vi "Main.vi"(8 "error in (no error)":errorcluster, 11 "BMCBase in":refnum<class "BMC.lvclass">) -> (0 "error out":errorcluster, 3 "component":refnum<class "BMC.lvclass">)   [LabVIEW 2012, in "BMC.lvclass"]
doc: "Main VI of the component."
uses:
  BMC.lvclass
  Murmex/LabVIEW/Murmex/Murmex/Murmex.lvclass
  Murmex/LabVIEW/Murmex/InitialiseMessage/InitialiseMessage.lvclass
  Murmex/LabVIEW/Murmex/TerminateMessage/TerminateMessage.lvclass
  Murmex/LabVIEW/Murmex/Message/Message.lvclass
  Murmex/LabVIEW/Murmex/ConfigureMessage/ConfigureMessage.lvclass
  Murmex/LabVIEW/Murmex/StartMessage/StartMessage.lvclass
  Murmex/LabVIEW/Murmex/StopMessage/StopMessage.lvclass
  Murmex/LabVIEW/Murmex/Murmex/update_cluster.ctl
  Murmex/LabVIEW/Murmex/Murmex/command_enum.ctl
  Controls/Voltage file.ctl
panel:
  in  "button::quit":bool
  in  "Tab Control":enum32{"Settings", "Debug"}(tab)
  in  "Multi mapping file":path=path "MultiMap.txt"
  in  "Voltage file":T1=path "MultiMap.txt"
  in  "button::configure":bool
  in  "button::start":bool
  in  "button::stop":bool
  in  "command":T2
  in  "button::send":bool
  in  "id":string="myself"
  out "Log":string
  in  "Generic command":string
  out "terminate?":bool
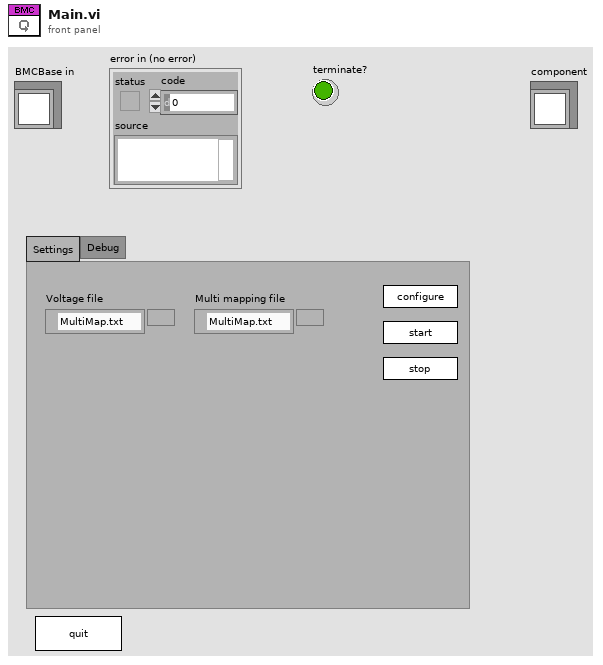
[diagram p1: front panel]
types:
  T1 = typedef "Voltage file.ctl" = path
  T2 = typedef "Murmex.lvclass/command_enum.ctl" = enum16{"null", "initialise", "reset", "terminate", "acknowledge", "update", "inspect", "inform", "proceed", "start", "stop", "fetch", "configure", "generic"}
  T3 = enum8{"Enabled", "Disabled", "Disabled and Grayed Out"}
  T4 = typedef "Murmex.lvclass/update_cluster.ctl" = cluster{"target ID":string, "key chains":string[], "values":variant[]}
  T5 = typedef "Murmex.lvclass/Event type enumerations.ctl" = enum16{"before", "after"}
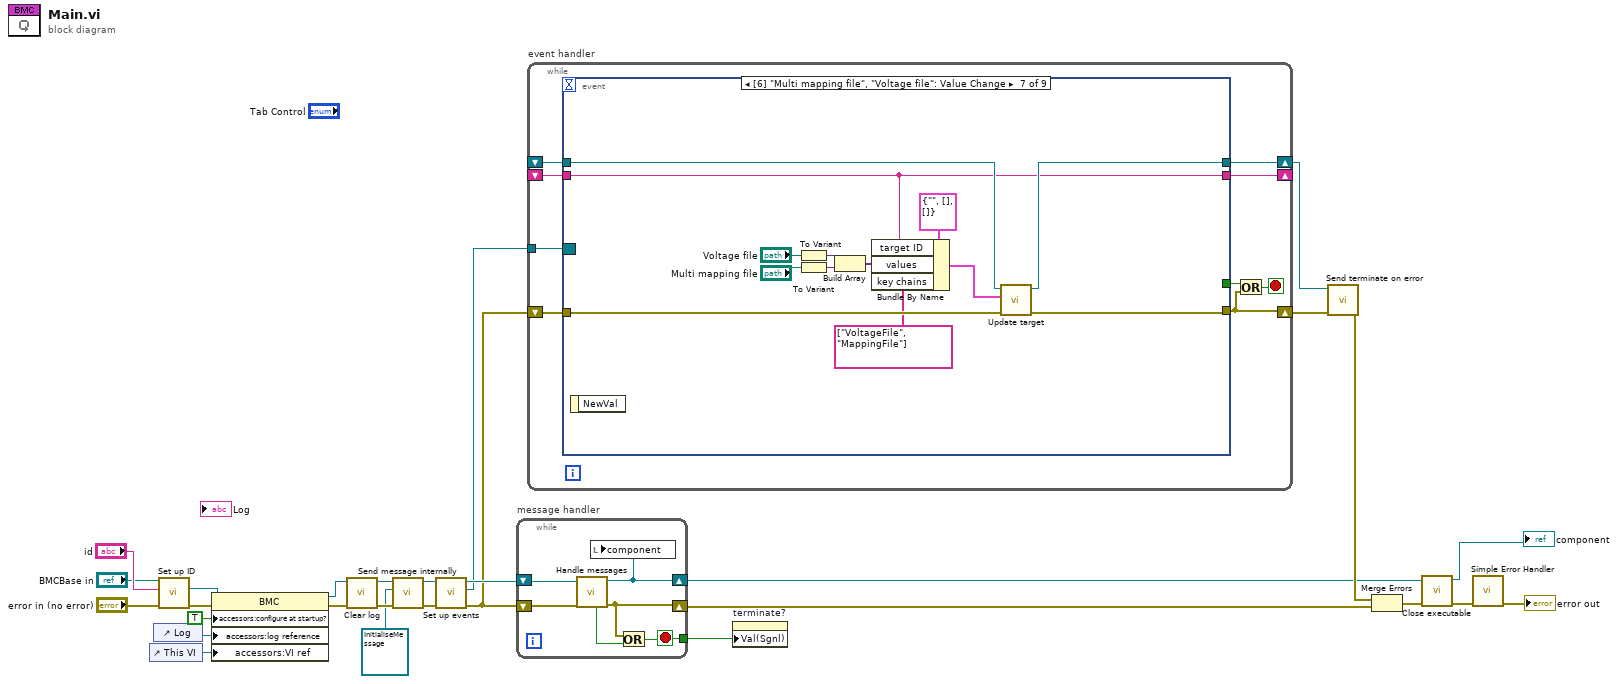
[diagram p0: block diagram]
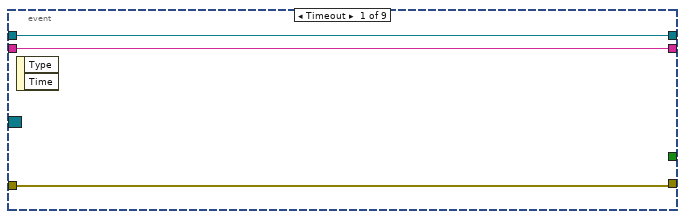
[diagram p2: hidden frame]
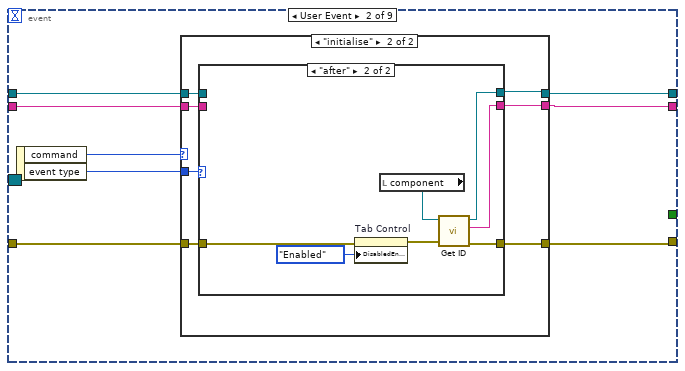
[diagram p3: hidden frame]
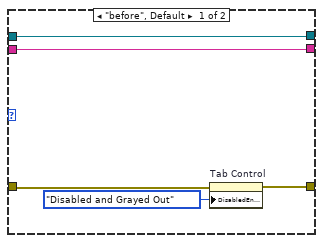
[diagram p5: hidden frame]
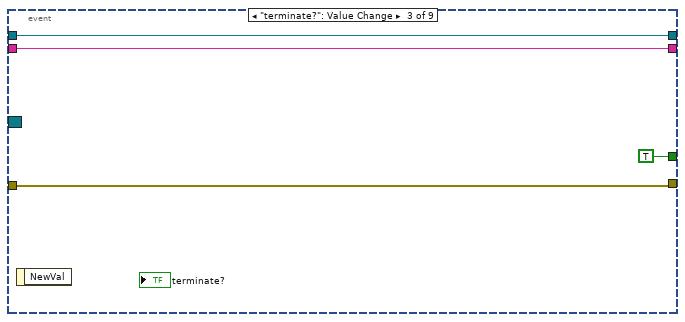
[diagram p6: hidden frame]
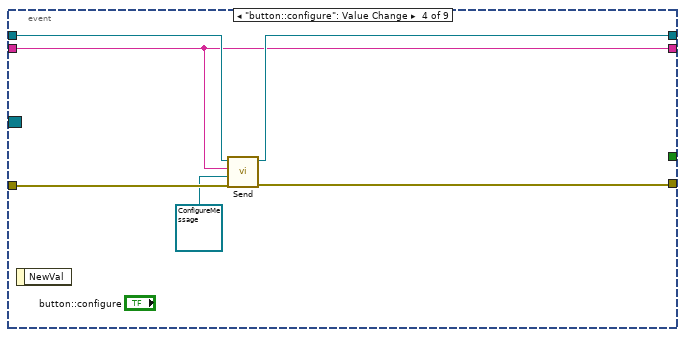
[diagram p7: hidden frame]
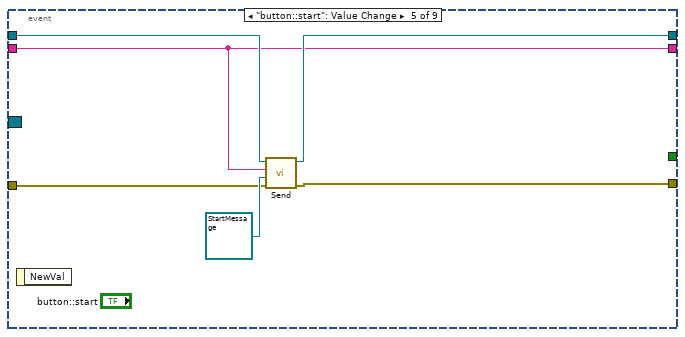
[diagram p8: hidden frame]
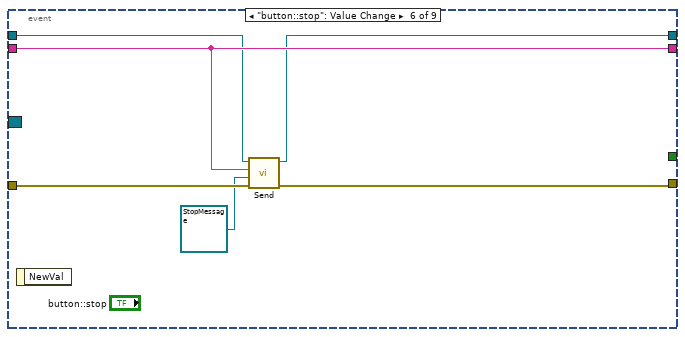
[diagram p9: hidden frame]
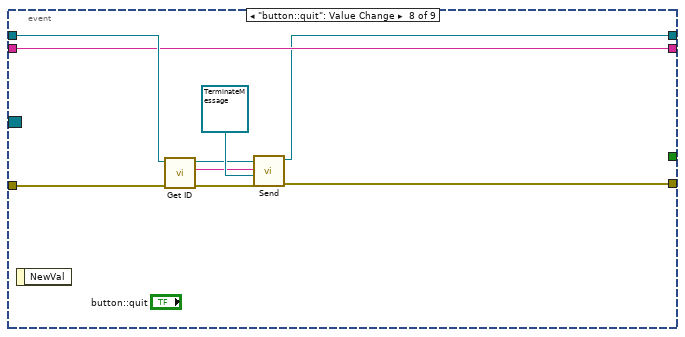
[diagram p10: hidden frame]
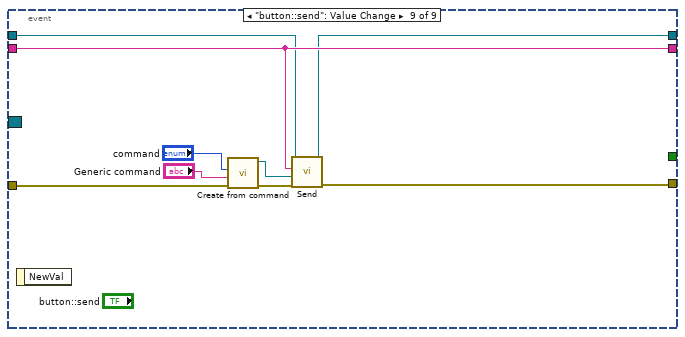
[diagram p11: hidden frame]
diagram:
  n1 = control-ref of="This VI"() -> (w22:refnum<vi>)
  n2 = control-ref of="Log"() -> (w21:refnum<vi>)
  n3 = call "Set up ID.vi"("error in (no error)"="error in (no error)", "component ID"="id", "MurmexBase in"="BMCBase in") -> ("error out"=w25:errorcluster, "MurmexBase out"=w24:refnum<class "BMC.lvclass">)  [unwired: 6 in, 1 out]
  n4 = property class="BMC"(reference=w24, error in=w25, "accessors:configure at startup?"=TRUE ("configure at startup?"), "accessors:log reference"=w21, "accessors:VI ref"=w22) -> (reference out=w17:refnum<class "BMC.lvclass">, error out=w20:errorcluster)
  n5 = call "Clear log.vi"("error in (no error)"=w20, "MurmexBase in"=w17) -> ("error out"=w19:errorcluster, "MurmexBase out"=w18:refnum<class "BMC.lvclass">)  [unwired: 8 in]
  n6 = call "Send message internally.vi"("error in (no error)"=w19, "Message"=refnum<class "InitialiseMessage.lvclass"> refnum ("InitialiseMessage"), "Murmex in"=w18) -> ("error out"=w15:errorcluster, "Murmex out"=w14:refnum<class "BMC.lvclass">)  [unwired: 7 in]
  n7 = call "Set up events.vi"("error in (no error)"=w15, "MurmexBase in"=w14) -> ("error out"=w6:errorcluster, "Event Registration Refnum"=w7:refnum<event-registration>, "MurmexBase out"=w13:refnum<class "BMC.lvclass">)  [unwired: 7 in]
  n8 = while "message handler" {
    shift-right: [w32] -> w8
    shift-left: w6 -> [w34]
    shift-right: [w29] -> w3
    shift-left: w13 -> [w33]
    tunnel: [w30] -> w12
    stop <- w30 stop-if-true
    n9 = call "Handle messages.vi"("error in (no error)"=w34, "Murmex in"=w33) -> ("error out"=w32:errorcluster, "Murmex out"=w29:refnum<class "BMC.lvclass">, "terminated?"=w31:bool)  [unwired: 7 in]
    n10 = local write "component"(w29) -> ()
    n11 = Or(x=w32, y=w31) -> (x .or. y?=w30:bool)
  }
  n12 = while "event handler" {
    tunnel: w7 -> [w41]
    shift-right: [w35] -> w5
    shift-left: w6 -> [w36]
    shift-right: [w40] -> w1
    shift-left: _ -> [w39]
    shift-right: [w38] -> _
    shift-left: _ -> [w37]
    stop <- w43 stop-if-true
    n13 = event shown="[6] \"Multi mapping file\", \"Voltage file\": Value Change" {
      selector: w41 -> [_ _ _ _ _ _ _ _ _]
      dyn-events: _ -> [_ _ _ _ _ _ _ _ _]
      timeout: _ -> [_ _ _ _ _ _ _ _ _]
      tunnel: [_ _ TRUE _ _ _ _ _ _] -> w42
      tunnel: [w46 w52 w79 w82 w88 w93 w108 w112 w121] -> w40
      tunnel: w39 -> [w46 w51 w79 w83 w89 w94 w109 w114 w122]
      tunnel: [w45 w50 w78 w81 w87 w95 w106 w113 w123] -> w38
      tunnel: w37 -> [w45 w49 w78 w81 w87 w95 w106 w113 w123]
      tunnel: w36 -> [w44 w48 w77 w86 w91 w98 w111 w120 w129]
      tunnel: [w44 w47 w77 w85 w90 w97 w110 w118 w125] -> w35
      event Timeout {
        n14 = event-data() -> ()  [unwired: 1 in, 2 out]
      }
      event User Event {
        n15 = event-data() -> ("command"=w54:T2, "event type"=w53:T5)  [unwired: 1 in]
        n16 = case shown="\"initialise\"" w54 {
          tunnel: w53 -> [_ w64]
          tunnel: [w56 w63] -> w52
          tunnel: w51 -> [w56 w62]
          tunnel: [w57 w61] -> w50
          tunnel: w49 -> [w57 w60]
          tunnel: w48 -> [w55 w59]
          tunnel: [w55 w58] -> w47
          frame "null", Default {
          }
          frame "initialise" {
            n17 = case shown="\"after\"" w64 {
              tunnel: [w68 w75] -> w63
              tunnel: w62 -> [w68 _]
              tunnel: [w67 w74] -> w61
              tunnel: w60 -> [w67 _]
              tunnel: w59 -> [w66 w70]
              tunnel: [w65 w71] -> w58
              frame "before", Default {
                n18 = property on="Tab Control" class="TabCtl (strict)"(error in=w66, "DisabledEnum"=T3."Disabled and Grayed Out" ("Disabled")) -> (error out=w65:errorcluster)  [unwired: 1 in, 1 out]
              }
              frame "after" {
                n19 = property on="Tab Control" class="TabCtl (strict)"(error in=w70, "DisabledEnum"=T3."Enabled" ("Disabled")) -> (error out=w73:errorcluster)  [unwired: 1 in, 1 out]
                n20 = local read "component"() -> (w76:refnum<class "BMC.lvclass">)
                n21 = call "Get ID.vi"("error in (no error)"=w73, "Murmex in"=w76) -> ("error out"=w71:errorcluster, "component id"=w74:string, "Murmex out"=w75:refnum<class "BMC.lvclass">)  [unwired: 7 in]
              }
            }
          }
        }
      }
      event "terminate?": Value Change {
        n22 = event-data() -> ()  [unwired: 1 in, 1 out]
      }
      event "button::configure": Value Change {
        n23 = event-data() -> ()  [unwired: 1 in, 1 out]
        n24 = call "Send.vi"("error in (no error)"=w86, "Message"=refnum<class "ConfigureMessage.lvclass"> refnum ("ConfigureMessage"), "recipient"=w81, "Murmex in"=w83) -> ("error out"=w85:errorcluster, "Murmex out"=w82:refnum<class "BMC.lvclass">)  [unwired: 6 in]
      }
      event "button::start": Value Change {
        n25 = event-data() -> ()  [unwired: 1 in, 1 out]
        n26 = call "Send.vi"("error in (no error)"=w91, "Message"=refnum<class "StartMessage.lvclass"> refnum ("StartMessage"), "recipient"=w87, "Murmex in"=w89) -> ("error out"=w90:errorcluster, "Murmex out"=w88:refnum<class "BMC.lvclass">)  [unwired: 6 in]
      }
      event "button::stop": Value Change {
        n27 = event-data() -> ()  [unwired: 1 in, 1 out]
        n28 = call "Send.vi"("error in (no error)"=w98, "Message"=refnum<class "StopMessage.lvclass"> refnum ("StopMessage"), "recipient"=w95, "Murmex in"=w94) -> ("error out"=w97:errorcluster, "Murmex out"=w93:refnum<class "BMC.lvclass">)  [unwired: 6 in]
      }
      event "Multi mapping file": Value Change {
        n29 = event-data() -> ()  [unwired: 1 in, 1 out]
        n30 = To Variant(anything="Voltage file") -> (Variant=w103:variant)
        n31 = To Variant(anything="Multi mapping file") -> (Variant=w102:variant)
        n32 = Build Array(w103, w102) -> (w104:variant[])
        n33 = Bundle By Name(cluster=T4 {"target ID"="", "key chains"=[], "values"=[]} ("update cluster"), "target ID"=w106, "values"=w104, "key chains"=string[] ["VoltageFile", "MappingFile"]) -> (w105:T4)
        n34 = call "Update target.vi"("error in (no error)"=w111, "update cluster"=w105, "MurmexBase in"=w109) -> ("error out"=w110:errorcluster, "MurmexBase out"=w108:refnum<class "BMC.lvclass">)  [unwired: 7 in]
      }
      event "button::quit": Value Change {
        n35 = event-data() -> ()  [unwired: 1 in, 1 out]
        n36 = call "Get ID.vi"("error in (no error)"=w120, "Murmex in"=w114) -> ("error out"=w119:errorcluster, "component id"=w115:string, "Murmex out"=w116:refnum<class "BMC.lvclass">)  [unwired: 7 in]
        n37 = call "Send.vi"("error in (no error)"=w119, "Message"=refnum<class "TerminateMessage.lvclass"> refnum ("TerminateMessage"), "recipient"=w115, "Murmex in"=w116) -> ("error out"=w118:errorcluster, "Murmex out"=w112:refnum<class "BMC.lvclass">)  [unwired: 6 in]
      }
      event "button::send": Value Change {
        n38 = event-data() -> ()  [unwired: 1 in, 1 out]
        n39 = call "Create from command.vi"("error in (no error)"=w129, "generic command"="Generic command", "command"="command") -> ("error out"=w126:errorcluster, "Message out"=w124:refnum<class "Message.lvclass">)  [unwired: 7 in]
        n40 = call "Send.vi"("error in (no error)"=w126, "Message"=w124, "recipient"=w123, "Murmex in"=w122) -> ("error out"=w125:errorcluster, "Murmex out"=w121:refnum<class "BMC.lvclass">)  [unwired: 6 in]
      }
    }
    n41 = Or(x=w42, y=w35) -> (x .or. y?=w43:bool)
  }
  n42 = property on="terminate?" class="Bool (strict)"("Val(Sgnl)"=w12) -> ()  [unwired: 2 in, 2 out]
  n43 = call "Send terminate on error.vi"("error in (no error)"=w5, "Murmex in"=w1) -> ("error out"=w4:errorcluster)  [unwired: 8 in, 1 out]
  n44 = Merge Errors(w4, w8) -> (w11:errorcluster)
  n45 = call "Close executable.vi"("error in (no error)"=w11, "MurmexBase in"=w3) -> ("error out"=w10:errorcluster, "MurmexBase out"=→"component":refnum<class "BMC.lvclass">)  [unwired: 8 in]
  n46 = call <vilib>:"Simple Error Handler.vi"("error in (no error)"=w10) -> ("error out"=→"error out":errorcluster)  [unwired: 4 in, 4 out]
